vi "HiFiveUnmatched_MakeChannel.vi"(7 "Sampling Rate [Hz]":dbl, 8 "Input Error":errorcluster, 10 "Input Task":refnum<k21>, 11 "Power Line Configurations":T1[](array[typedef])) -> (0 "Output Error":errorcluster, 3 "Output Task":refnum<k21>)   [LabVIEW 2020]
uses:
  HiFiveUnmatched_PowerLineCfg.ctl
  <vilib>/DAQmx/create/channels.llb/DAQmx Create Channel (AI-Current-Basic).vi
  <vilib>/DAQmx/configure/timing.llb/DAQmx Timing (Sample Clock).vi
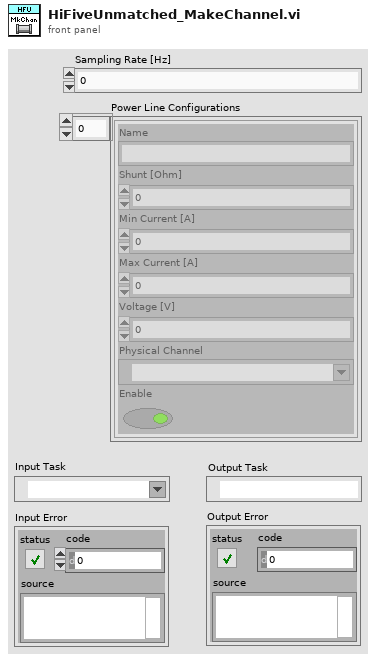
[diagram p1: front panel]
types:
  T1 = typedef "HiFiveUnmatched_PowerLineCfg.ctl" = cluster{"Name":string, "Shunt [Ohm]":dbl, "Min Current [A]":dbl, "Max Current [A]":dbl, "Voltage [V]":dbl, "Physical Channel":tag, "Enable":bool}
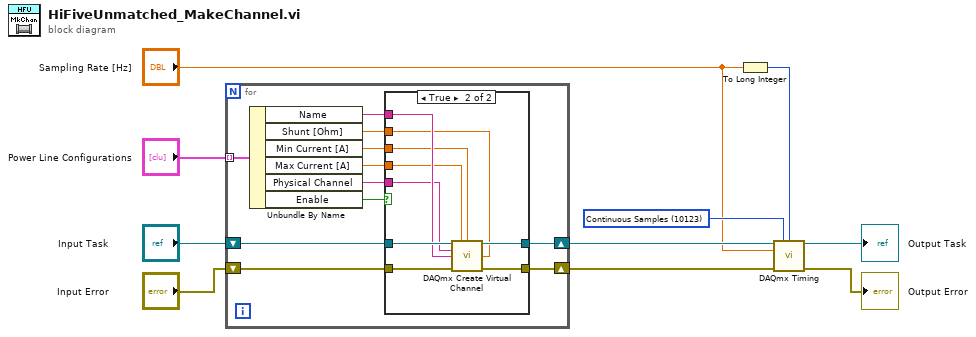
[diagram p0: block diagram]
diagram:
  w7 = 10123 items=["Finite Samples"=10178, "Continuous Samples"=10123, "Hardware Timed Single Point"=12522] ("sample mode")
  n1 = for {
    shift-right: [w20] -> w5
    shift-left: "Input Task" -> [w18]
    shift-right: [w21] -> w4
    shift-left: "Input Error" -> [w19]
    tunnel: "Power Line Configurations" -> [w17] mode=indexing
    n2 = Unbundle By Name(w17) -> ("Name"=w11:string, "Shunt [Ohm]"=w12:dbl, "Min Current [A]"=w13:dbl, "Max Current [A]"=w14:dbl, "Physical Channel"=w15:tag, "Enable"=w16:bool)
    n3 = case shown="True" w16 {
      tunnel: [w23 w32] -> w21
      tunnel: [w22 w31] -> w20
      tunnel: w19 -> [w23 w30]
      tunnel: w18 -> [w22 w29]
      tunnel: w15 -> [_ w24]
      tunnel: w14 -> [_ w25]
      tunnel: w13 -> [_ w26]
      tunnel: w12 -> [_ w27]
      tunnel: w11 -> [_ w28]
      frame False {
      }
      frame True {
        n4 = call-poly <vilib>:"DAQmx Create Virtual Channel.vi"("task in"=w29, "maximum value"=w25, "minimum value"=w26, "physical channels"=w24, "name to assign"=w28, "external shunt resistor value"=w27, "error in"=w30) -> ("task out"=w31:refnum<k21>, "error out"=w32:errorcluster)  [unwired: 7 in]
      }
    }
  }
  n5 = To Long Integer(number="Sampling Rate [Hz]") -> (32bit integer=w6:i32)
  n6 = call-poly <vilib>:"DAQmx Timing.vi"("task/channels in"=w5, "sample mode"=w7, "samples per channel"=w6, "rate"="Sampling Rate [Hz]", "error in"=w4) -> ("task out"=→"Output Task":refnum<k21>, "error out"=→"Output Error":errorcluster)  [unwired: 9 in]
